vi "Server Loop Async.vi"(11 "TCP Server in":refnum<class "TCP Server.lvclass">) -> ()   [LabVIEW 2020, in "Stream-TCP.lvlib" / "TCP Server.lvclass"]
uses:
  TCP Server.lvclass
  C:/Program Files (x86)/National Instruments/LabVIEW 2020/vi.lib/IlluminatedG/lv-stream/Endpoint/Endpoint.lvclass
  <vilib>/IlluminatedG/lv-stream/Endpoint/Endpoint.lvclass
  TCP Server.lvclass/TCP Server.ctl
  TCP Client/TCP Client.lvclass
panel:
  out "URI String":string
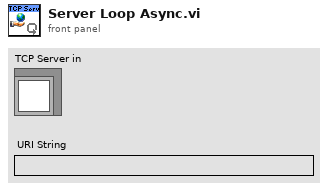
[diagram p1: front panel]
types:
  T1 = typedef "Stream-TCP.lvlib/Listener Notifier.ctl" = refnum<notifier>
  T2 = typedef "Stream-TCP.lvlib/Listener Result.ctl" = cluster{"Status":T3, "Client":refnum<class "TCP Client.lvclass">, "Ack Notifier":refnum<notifier>}
  T3 = typedef "Stream-TCP.lvlib/Listener Status.ctl" = enum16{"Successful", "Unsuccessful"}
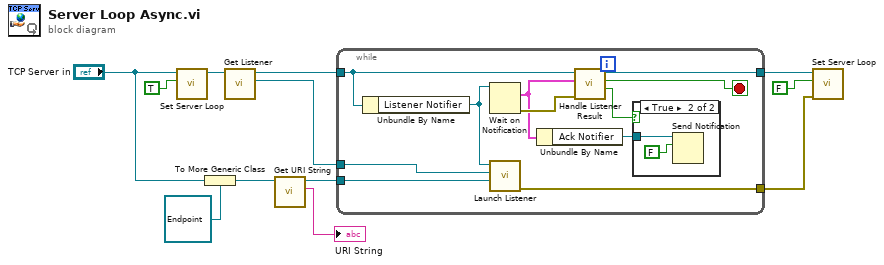
[diagram p0: block diagram]
diagram:
  n1 = call "Set Server Loop.vi"("Server Loop"=TRUE, "TCP Server in"="TCP Server in") -> ("TCP Server out"=w6:refnum<class "TCP Server.lvclass">)  [unwired: 8 in, 1 out]
  n2 = To More Generic Class(target class=refnum<class "Endpoint.lvclass"> refnum ("Stream.lvlib:Endpoint.lvclass"), reference="TCP Server in") -> (generic class reference=w10:refnum<class "Endpoint.lvclass">)
  n3 = call "Get Listener.vi"("TCP Server in"=w6) -> ("Listener"=w7:refnum<k5>, "TCP Server out"=w4:refnum<class "TCP Server.lvclass">)  [unwired: 8 in, 1 out]
  n4 = call <vilib>:"Get URI String.vi"("Endpoint in"=w10) -> ("URI String"=→"URI String":string, "Endpoint out"=w8:refnum<class "Endpoint.lvclass">)  [unwired: 8 in, 1 out]
  n5 = while {
    tunnel: w7 -> [w19]
    tunnel: w8 -> [w17]
    tunnel: [w21] -> w3
    tunnel: w4 -> [w20]
    tunnel: [w16] -> w1
    stop <- w23 stop-if-true
    n6 = Unbundle By Name(w20) -> ("Listener Notifier"=w18:T1)
    n7 = Wait on Notification(notifier=w18) -> (notification=w15:T2, error out=w22:errorcluster)  [unwired: 3 in, 2 out]
    n8 = call "Launch Listener.vi"("Endpoint"=w17, "Listener"=w19, "Listener Notifier"=w18) -> ("error out"=w16:errorcluster)  [unwired: 8 in]
    n9 = Unbundle By Name(w15) -> ("Ack Notifier"=w13:refnum<notifier>)
    n10 = call "Handle Listener Result.vi"("error in (no error)"=w22, "Result"=w15, "TCP Server in"=w20) -> ("Send Ack"=w14:bool, "Shutdown"=w23:bool, "TCP Server out"=w21:refnum<class "TCP Server.lvclass">)  [unwired: 5 in, 1 out]
    n11 = case shown="True" w14 {
      tunnel: w13 -> [_ w25]
      frame False {
      }
      frame True {
        n12 = Send Notification(notification=FALSE, notifier=w25) -> ()  [unwired: 1 in, 2 out]
      }
    }
  }
  n13 = call "Set Server Loop.vi"("error in (no error)"=w1, "Server Loop"=FALSE, "TCP Server in"=w3) -> ()  [unwired: 7 in, 2 out]
